vi "Telnet Create Connection.vi"(8 "error in (no error)":errorcluster, 11 "TCP connection":refnum<k5>) -> (0 "error out":errorcluster, 3 "telnet connection":T3)   [LabVIEW 2014]
doc: "Opens a Telnet connection."
uses:
  Telnet Session.ctl
  Telnet Connection Data.ctl
  Semaphore RefNum.ctl
panel:
  in  "not a refnum error":errorcluster={"status"=TRUE, "code"=1000, "source"="Telnet Create Connection:\nnot a valid TCP connection"}
  in  "telnet data":T1
  in  "empty object":T3
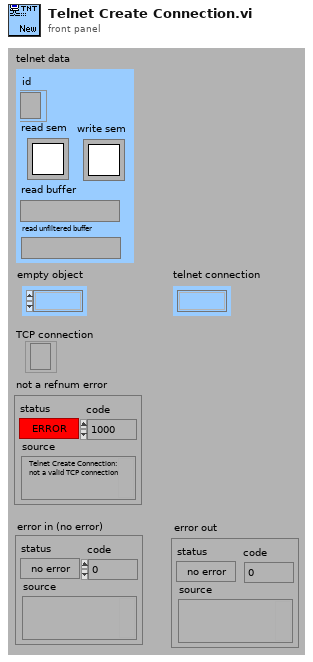
[diagram p1: front panel]
types:
  T1 = typedef "Telnet Connection Data.ctl" = cluster{"id":refnum<k5>, "read sem":T2, "write sem":T2, "read buffer":string, "read unfiltered buffer":string}
  T2 = typedef "Semaphore RefNum.ctl" = refnum<k1>
  T3 = typedef "Telnet Session.ctl" = refnum<k1>
  T4 = enum16{"reset", "register", "get data", "set data", "unregister", "test", "get objects"}
  T5 = typedef "Semaphore RefNum" = refnum<k1>
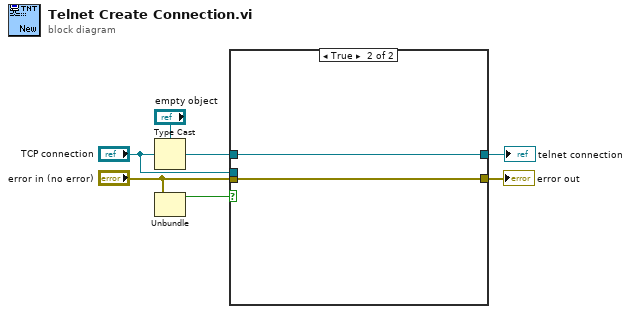
[diagram p0: block diagram]
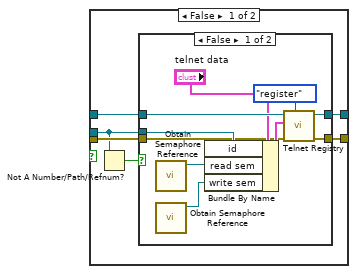
[diagram p2: hidden frame]
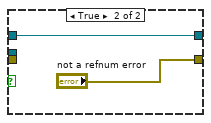
[diagram p3: hidden frame]
diagram:
  n1 = Type Cast(type="empty object", x="TCP connection") -> (*(type *) &x=w4:T3)
  n2 = Unbundle("error in (no error)") -> ("status"=w3:bool)  [unwired: 2 out]
  n3 = case shown="True" w3 {
    tunnel: "error in (no error)" -> [w13 w27]
    tunnel: w4 -> [w10 w26]
    tunnel: [w12 w26] -> w6
    tunnel: [w11 w27] -> w7
    tunnel: "TCP connection" -> [w9 _]
    frame False {
      n4 = Not A Number/Path/Refnum?(number/path/refnum=w9) -> (NaN/Path/Refnum?=w8:bool)
      n5 = case shown="False" w8 {
        tunnel: w9 -> [w21 _]
        tunnel: w10 -> [w20 w25]
        tunnel: [w17 "not a refnum error"] -> w11
        tunnel: [w16 w25] -> w12
        tunnel: w13 -> [w14 _]
        frame False {
          n6 = call <vilib>:"Obtain Semaphore Reference.vi"() -> ("semaphore"=w22:T5)  [unwired: 5 in, 2 out]
          n7 = call <vilib>:"Obtain Semaphore Reference.vi"() -> ("semaphore"=w23:T5)  [unwired: 5 in, 2 out]
          n8 = Bundle By Name(cluster="telnet data", "id"=w21, "read sem"=w22, "write sem"=w23) -> (w19:T1)
          n9 = call "Telnet Registry.vi"("function (get data)"=T4."register", "error in (no error)"=w14, "object data in"=w19, "object"=w20) -> ("error out"=w17:errorcluster, "object out"=w16:T3)  [unwired: 3 in, 3 out]
        }
        frame True {
        }
      }
    }
    frame True {
    }
  }
  "error out" <- w7
  "telnet connection" <- w6
